vi "main.vi"() -> ()   [LabVIEW 2020]
uses:
  Typedef/QueueOperation.ctl
  Typedef/TimeCluster.ctl
  Strict Type Def/LowBean.ctl
  Strict Type Def/LowMilk.ctl
  Strict Type Def/Chamber.ctl
  Strict Type Def/Dispenser.ctl
  Strict Type Def/Low Water.ctl
  Strict Type Def/Purging.ctl
  Strict Type Def/Heating.ctl
  Strict Type Def/Grinding.ctl
  Strict Type Def/Brewing.ctl
  Strict Type Def/Dispensing.ctl
  Typedef/DataCluster.ctl
  <vilib>/Utility/config.llb/NI_LVConfig.lvlib
panel:
  out "error out":errorcluster
  in  "error in (no error)":errorcluster
  in  "Power":bool
  out "Total Cups":i32
  out "Elapsed Time":dbl
  out "Dispensing":T1
  out "Brewing":T2
  out "Grinding":T3
  out "Heating":T4
  out "Purging":T5
  out "Dispenser":T6 scale=0.0..60.0
  out "Chamber":T7 scale=0.0..60.0
  out "Low Milk":T8
  out "Low Bean":T9
  out "Low Water":T10
  out "Milk Level":i32(slide) min=0 max=100 scale=0.0..100.0
  out "Bean Level":i32(slide) min=0 max=100 scale=0.0..100.0
  out "Water Level":i32(slide) min=0 max=100 scale=0.0..100.0
  in  "Type":i32(knob) scale=0.0..2.0
  in  "Carafe":bool
  in  "Cup":bool
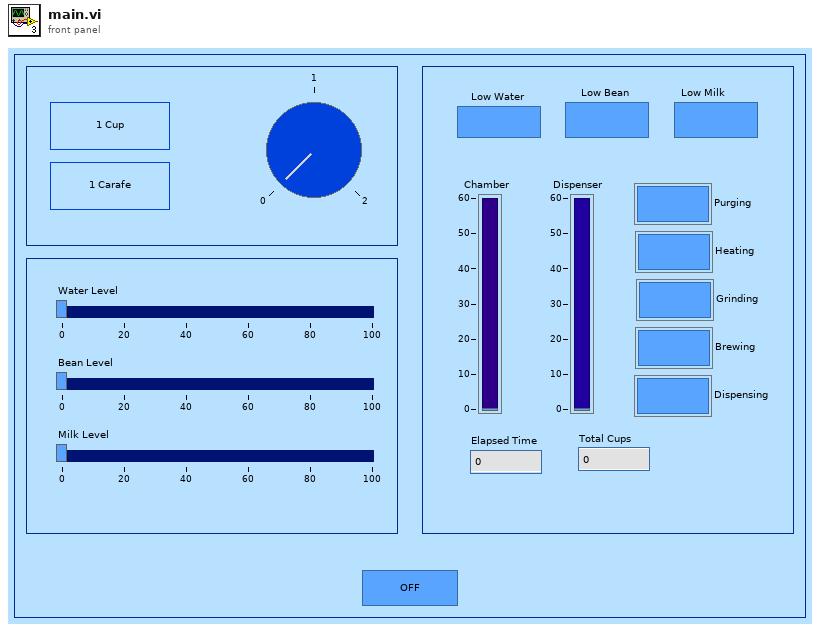
[diagram p1: front panel]
types:
  T1 = typedef "Dispensing.ctl" = bool
  T2 = typedef "Brewing.ctl" = bool
  T3 = typedef "Grinding.ctl" = bool
  T4 = typedef "Heating.ctl" = bool
  T5 = typedef "Purging.ctl" = bool
  T6 = typedef "Dispenser.ctl" = u8
  T7 = typedef "Chamber.ctl" = u8
  T8 = typedef "LowMilk.ctl" = bool
  T9 = typedef "LowBean.ctl" = bool
  T10 = typedef "Low Water.ctl" = bool
  T11 = typedef "DataCluster.ctl" = cluster{"Cup":bool, "Type":i32, "Carafe":bool, "Bean Level":i32, "Water Level":i32, "Milk Level":i32, "Low Bean":T9, "Low Milk":T8, "Chamber":T7, "Dispenser":T6, "Low Water":T10, "Elapsed Time":dbl, "Purging":T5, "Heating":T4, "Grinding":T3, "Brewing":T2, "Dispensing":T1, "Total Cups":i32, "Power":bool, "Timer":T12, "Path":path, "Shutdown":bool}
  T12 = typedef "TimeCluster.ctl" = cluster{"Relative time":dbl, "Initial Time":dbl, "Set Timer":i32, "Start/Stop":bool, "Pause/Resume":bool}
  T13 = typedef "QueueOperation.ctl" = enum16{"Create", "Enqueue", "Dequeue", "Flush", "Close"}
  T14 = enum8{"Enabled", "Disabled", "Disabled and Grayed Out"}
  T15 = typedef "NI_LVConfig.lvlib/Config Data RefNum.ctl" = refnum<k1>
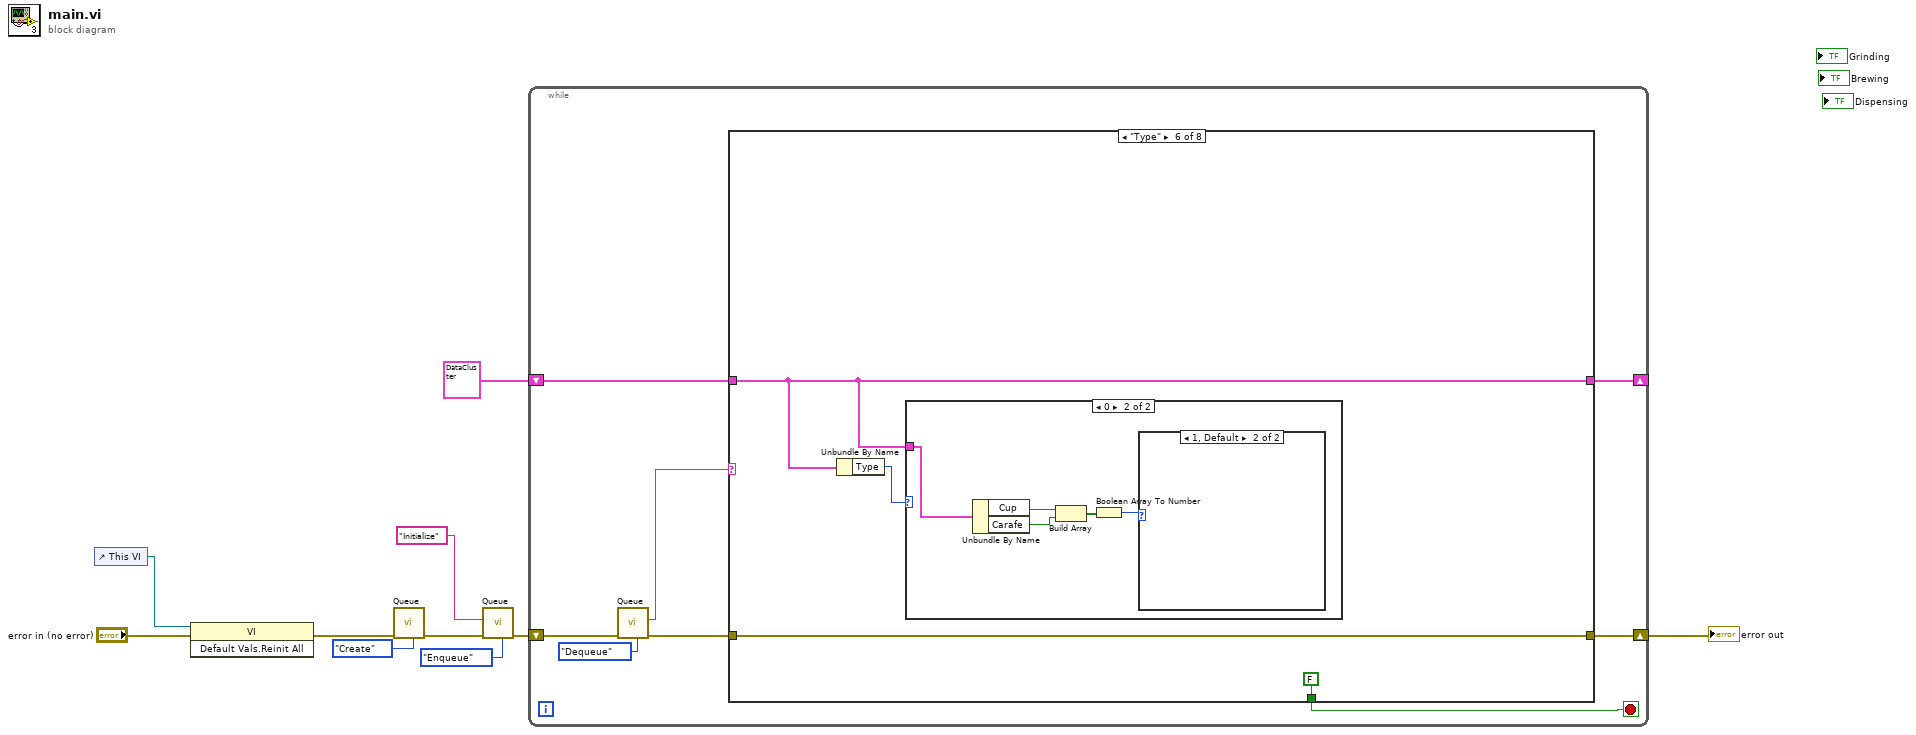
[diagram p0: block diagram]
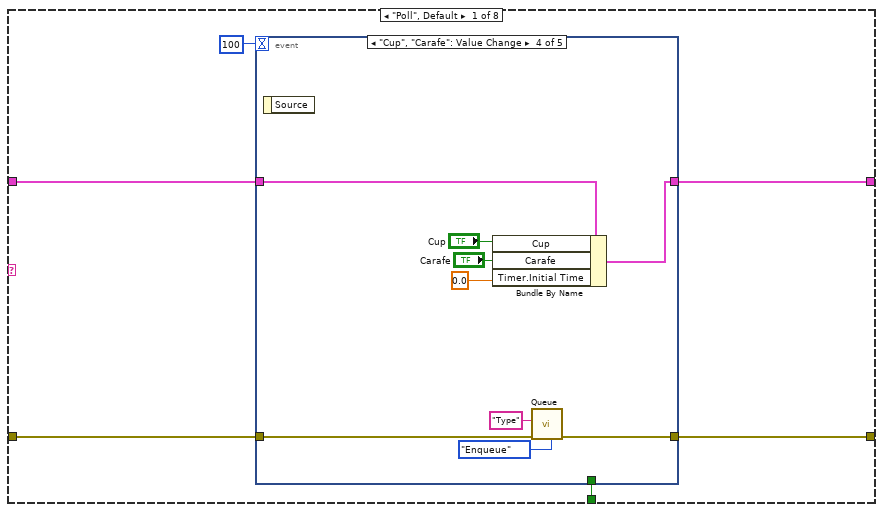
[diagram p2: hidden frame]
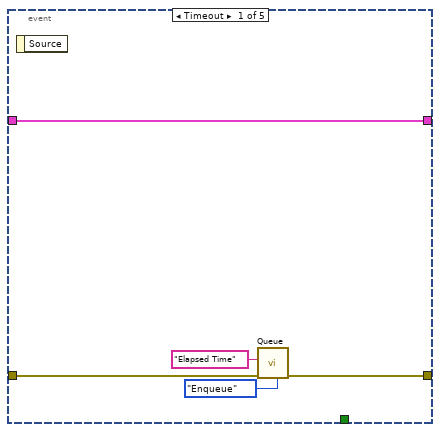
[diagram p3: hidden frame]
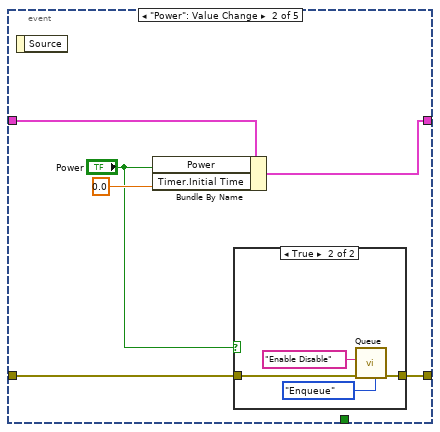
[diagram p4: hidden frame]
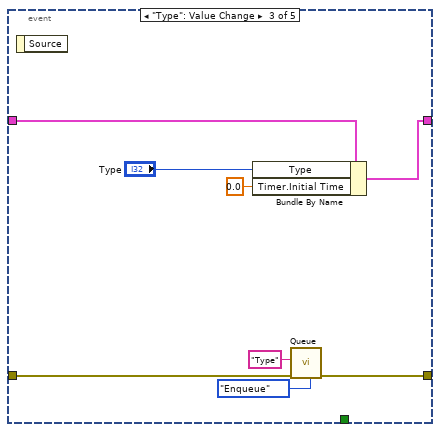
[diagram p6: hidden frame]
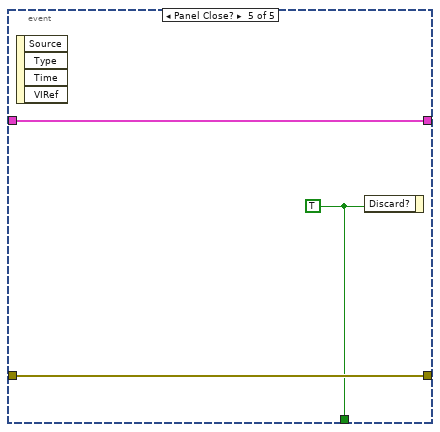
[diagram p7: hidden frame]
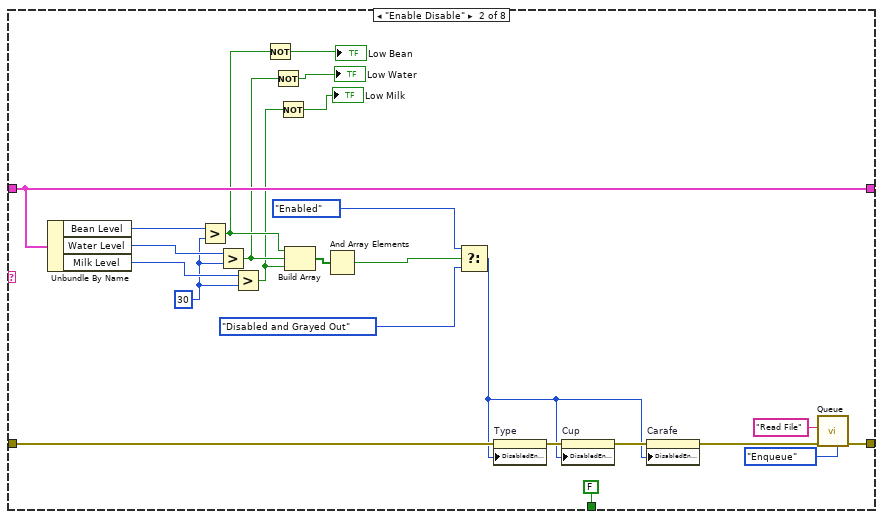
[diagram p8: hidden frame]
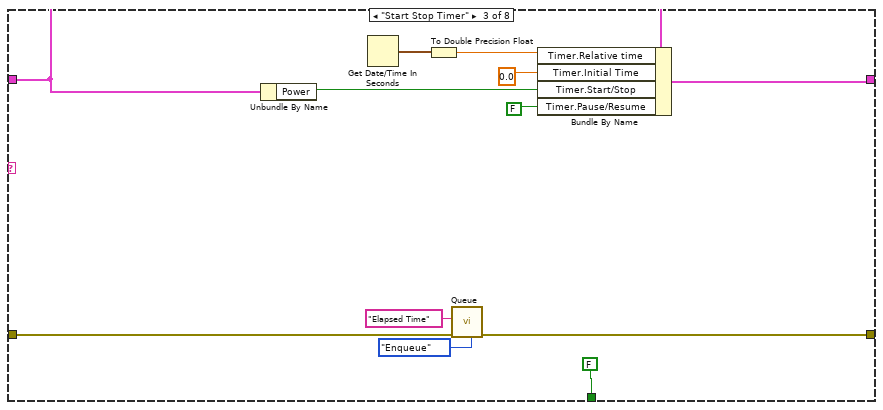
[diagram p9: hidden frame]
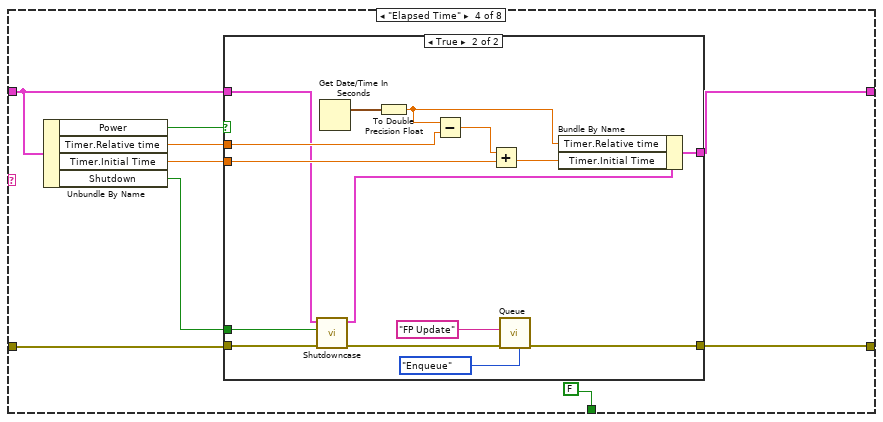
[diagram p10: hidden frame]
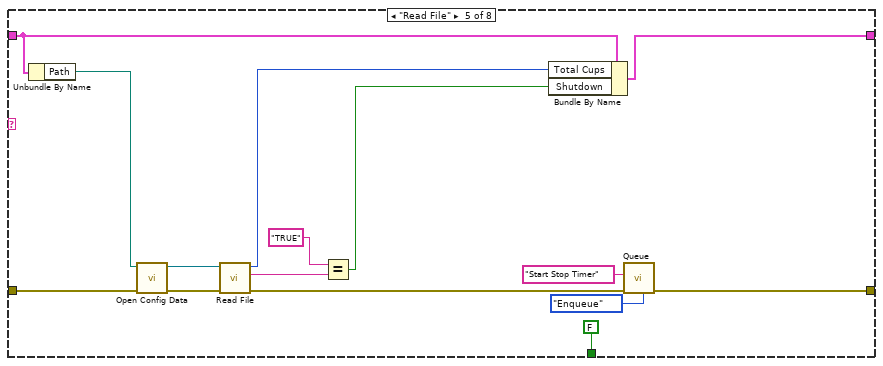
[diagram p12: hidden frame]
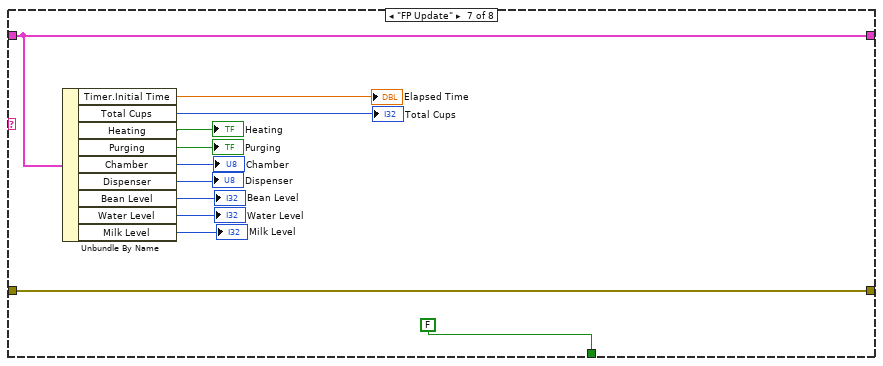
[diagram p15: hidden frame]
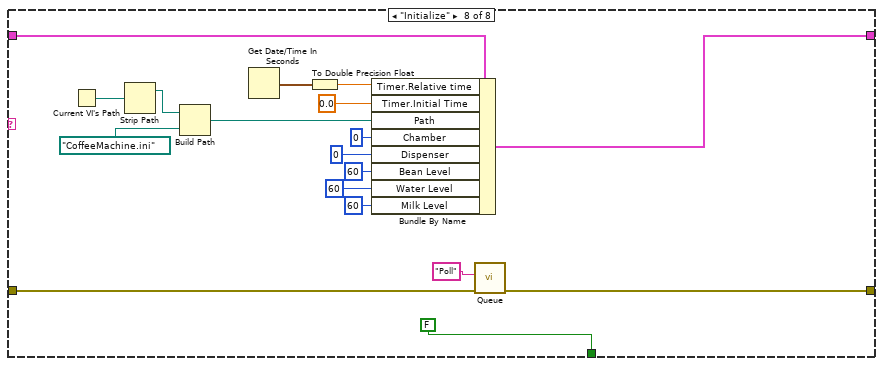
[diagram p16: hidden frame]
diagram:
  n1 = control-ref of="This VI"() -> (w8:refnum<vi>)
  n2 = invoke class="VI" method="Default Vals.Reinit All"(reference=w8, error in="error in (no error)") -> (error out=w7:errorcluster)  [unwired: 1 in, 2 out]
  n3 = call "Queue.vi"("Enum"=QueueOperation."Create", "error in (no error)"=w7) -> ("error out"=w5:errorcluster)  [unwired: 7 in, 2 out]
  n4 = call "Queue.vi"("Enum"=QueueOperation."Enqueue", "error in (no error)"=w5, "Enqueue Element"="Initialize") -> ("error out"=w4:errorcluster)  [unwired: 6 in, 2 out]
  n5 = while {
    shift-right: [w16] -> w9
    shift-left: w4 -> [w18]
    shift-right: [w13] -> _
    shift-left: T11 {"Cup"=FALSE, "Type"=0, "Carafe"=FALSE, "Bean Level"=0, "Water Level"=0, "Milk Level"=0, "Low Bean"=FALSE, "Low Milk"=FALSE, "Chamber"=1, "Dispenser"=1, "Low Water"=FALSE, "Elapsed Time"=0.0, "Purging"=FALSE, "Heating"=FALSE, "Grinding"=FALSE, "Brewing"=FALSE, "Dispensing"=FALSE, "Total Cups"=0, "Power"=FALSE, "Timer"={"Relative time"=0.0, "Initial Time"=0.0, "Set Timer"=0, "Start/Stop"=FALSE, "Pause/Resume"=FALSE}, "Path"=path "", "Shutdown"=FALSE} -> [w12]
    stop <- w11 stop-if-true
    n6 = call "Queue.vi"("Enum"=QueueOperation."Dequeue", "error in (no error)"=w18) -> ("error out"=w15:errorcluster, "Dequeued Element"=w14:string)  [unwired: 7 in, 1 out]
    n7 = case shown="\"Type\"" w14 {
      tunnel: [w24 w72 w87 w100 w125 w141 w158 w175] -> w16
      tunnel: w15 -> [w23 w84 w88 w99 w136 w141 w158 w176]
      tunnel: [w21 w82 w96 w101 w128 w138 w156 w171] -> w13
      tunnel: w12 -> [w20 w82 w90 w102 w129 w138 w156 w172]
      tunnel: [w19 FALSE FALSE FALSE FALSE FALSE FALSE FALSE] -> w11
      frame "Poll", Default {
        n8 = event shown="[3] \"Cup\", \"Carafe\": Value Change" {
          selector: _ -> [_ _ _ _ _]
          dyn-events: _ -> [_ _ _ _ _]
          timeout: 100 -> [_ _ _ _ _]
          tunnel: [w27 w32 w43 w52 w59] -> w24
          tunnel: w23 -> [w28 w33 w44 w53 w59]
          tunnel: [w29 w34 w47 w57 w60] -> w21
          tunnel: w20 -> [w29 w35 w48 w51 w60]
          tunnel: [_ _ _ _ w58] -> w19
          event Timeout {
            n9 = event-data() -> ()  [unwired: 1 in, 1 out]
            n10 = call "Queue.vi"("Enum"=QueueOperation."Enqueue", "error in (no error)"=w28, "Enqueue Element"="Elapsed Time") -> ("error out"=w27:errorcluster)  [unwired: 6 in, 2 out]
          }
          event "Power": Value Change {
            n11 = event-data() -> ()  [unwired: 1 in, 1 out]
            n12 = Bundle By Name(cluster=w35, "Power"="Power", "Timer.Initial Time"=0.0) -> (w34:T11)
            n13 = case shown="True" "Power" {
              tunnel: w33 -> [w36 w40]
              tunnel: [w36 w39] -> w32
              frame False {
              }
              frame True {
                n14 = call "Queue.vi"("Enum"=QueueOperation."Enqueue", "error in (no error)"=w40, "Enqueue Element"="Enable Disable") -> ("error out"=w39:errorcluster)  [unwired: 6 in, 2 out]
              }
            }
          }
          event "Type": Value Change {
            n15 = event-data() -> ()  [unwired: 1 in, 1 out]
            n16 = Bundle By Name(cluster=w48, "Type"="Type", "Timer.Initial Time"=0.0) -> (w47:T11)
            n17 = call "Queue.vi"("Enum"=QueueOperation."Enqueue", "error in (no error)"=w44, "Enqueue Element"="Type") -> ("error out"=w43:errorcluster)  [unwired: 6 in, 2 out]
          }
          event "Cup", "Carafe": Value Change {
            n18 = event-data() -> ()  [unwired: 1 in, 1 out]
            n19 = Bundle By Name(cluster=w51, "Cup"="Cup", "Carafe"="Carafe", "Timer.Initial Time"=0.0) -> (w57:T11)
            n20 = call "Queue.vi"("Enum"=QueueOperation."Enqueue", "error in (no error)"=w53, "Enqueue Element"="Type") -> ("error out"=w52:errorcluster)  [unwired: 6 in, 2 out]
          }
          event Panel Close? {
            w58 = TRUE
            n21 = event-data() -> ()  [unwired: 1 in, 4 out]
            n22 = event-data("Discard?"=w58) -> ()  [unwired: 1 in, 1 out]
          }
        }
      }
      frame "Enable Disable" {
        w78 = 30
        n23 = Unbundle By Name(w82) -> ("Bean Level"=w81:i32, "Water Level"=w80:i32, "Milk Level"=w79:i32)
        n24 = Greater?(x=w81, y=w78) -> (0:w65:bool)
        n25 = Greater?(x=w80, y=w78) -> (0:w63:bool)
        n26 = Greater?(x=w79, y=w78) -> (0:w61:bool)
        n27 = Not(x=w65) -> (.not. x?=→"Low Bean":bool)
        n28 = Not(x=w63) -> (.not. x?=→"Low Water":bool)
        n29 = Not(x=w61) -> (.not. x?=→"Low Milk":bool)
        n30 = Build Array(w65, w63, w61) -> (w77:bool[])
        n31 = And Array Elements(Boolean array=w77) -> (logical AND=w76:bool)
        n32 = Select(t=T14."Enabled" ("Disabled"), s=w76, f=T14."Disabled and Grayed Out" ("Disabled")) -> (s? t:f=w67:T14)
        n33 = property on="Type" class="Knob (strict)"(error in=w84, "DisabledEnum"=w67) -> (error out=w73:errorcluster)  [unwired: 1 in, 1 out]
        n34 = property on="Cup" class="Bool"(error in=w73, "DisabledEnum"=w67) -> (error out=w69:errorcluster)  [unwired: 1 in, 1 out]
        n35 = property on="Carafe" class="Bool"(error in=w69, "DisabledEnum"=w67) -> (error out=w68:errorcluster)  [unwired: 1 in, 1 out]
        n36 = call "Queue.vi"("Enum"=QueueOperation."Enqueue", "error in (no error)"=w68, "Enqueue Element"="Read File") -> ("error out"=w72:errorcluster)  [unwired: 6 in, 2 out]
      }
      frame "Start Stop Timer" {
        n37 = Unbundle By Name(w90) -> ("Power"=w89:bool)
        n38 = Get Date/Time In Seconds() -> (seconds since 1Jan1904=w95:timestamp)
        n39 = To Double Precision Float(number=w95) -> (double precision float=w94:dbl)
        n40 = call "Queue.vi"("Enum"=QueueOperation."Enqueue", "error in (no error)"=w88, "Enqueue Element"="Elapsed Time") -> ("error out"=w87:errorcluster)  [unwired: 6 in, 2 out]
        n41 = Bundle By Name(cluster=w90, "Timer.Relative time"=w94, "Timer.Initial Time"=0.0, "Timer.Start/Stop"=w89, "Timer.Pause/Resume"=FALSE) -> (w96:T11)
      }
      frame "Elapsed Time" {
        n42 = Unbundle By Name(w102) -> ("Power"=w98:bool, "Timer.Relative time"=w104:dbl, "Timer.Initial Time"=w103:dbl, "Shutdown"=w97:bool)
        n43 = case shown="True" w98 {
          tunnel: w104 -> [_ w122]
          tunnel: w103 -> [_ w121]
          tunnel: w102 -> [w107 w109]
          tunnel: [w107 w120] -> w101
          tunnel: [w106 w119] -> w100
          tunnel: w99 -> [w106 w116]
          tunnel: w97 -> [_ w110]
          frame False {
          }
          frame True {
            n44 = call "Shutdowncase.vi"("error in (no error)"=w116, "Boolean"=w110, "Data Cluster"=w109) -> ("error out"=w115:errorcluster, "output cluster"=w108:T11)  [unwired: 7 in]
            n45 = Get Date/Time In Seconds() -> (seconds since 1Jan1904=w114:timestamp)
            n46 = To Double Precision Float(number=w114) -> (double precision float=w112:dbl)
            n47 = Subtract(x=w112, y=w122) -> (x-y=w113:dbl)
            n48 = Add(x=w113, y=w121) -> (x+y=w111:dbl)
            n49 = call "Queue.vi"("Enum"=QueueOperation."Enqueue", "error in (no error)"=w115, "Enqueue Element"="FP Update") -> ("error out"=w119:errorcluster)  [unwired: 6 in, 2 out]
            n50 = Bundle By Name(cluster=w108, "Timer.Relative time"=w112, "Timer.Initial Time"=w111) -> (w120:T11)
          }
        }
      }
      frame "Read File" {
        n51 = Unbundle By Name(w129) -> ("Path"=w135:path)
        n52 = call <vilib>:"Open Config Data.vi"("error in (no error)"=w136, "configuration file path"=w135) -> ("error out"=w134:errorcluster, "refnum"=w133:T15)  [unwired: 7 in, 1 out]
        n53 = call "Read File.vi"("error in (no error)"=w134, "Refnum in"=w133) -> ("error out"=w126:errorcluster, "value"=w132:string, "value 2"=w130:i32)  [unwired: 7 in]
        n54 = Equal?(x="TRUE", y=w132) -> (x = y?=w127:bool)
        n55 = Bundle By Name(cluster=w129, "Total Cups"=w130, "Shutdown"=w127) -> (w128:T11)
        n56 = call "Queue.vi"("Enum"=QueueOperation."Enqueue", "error in (no error)"=w126, "Enqueue Element"="Start Stop Timer") -> ("error out"=w125:errorcluster)  [unwired: 6 in, 2 out]
      }
      frame "Type" {
        n57 = Unbundle By Name(w138) -> ("Type"=w139:i32)
        n58 = case shown="0" w139 {
          tunnel: w138 -> [_ w146]
          frame 0, Default {
          }
          frame 0 {
            n59 = Unbundle By Name(w146) -> ("Cup"=w145:bool, "Carafe"=w144:bool)
            n60 = Build Array(w145, w144) -> (w143:bool[])
            n61 = Boolean Array To Number(Boolean array=w143) -> (number=w142:u32)
            n62 = case shown="1, Default" w142 {
              frame 0 {
              }
              frame 1, Default {
              }
            }
          }
        }
      }
      frame "FP Update" {
        n63 = Unbundle By Name(w156) -> ("Timer.Initial Time"=→"Elapsed Time":dbl, "Total Cups"=→"Total Cups":i32, "Heating"=→"Heating":T4, "Purging"=→"Purging":T5, "Chamber"=→"Chamber":T7, "Dispenser"=→"Dispenser":T6, "Bean Level"=→"Bean Level":i32, "Water Level"=→"Water Level":i32, "Milk Level"=→"Milk Level":i32)
      }
      frame "Initialize" {
        n64 = Current VI's Path() -> (path=w167:path)
        n65 = Strip Path(path=w167) -> (stripped path=w166:path)  [unwired: 1 out]
        n66 = Build Path(base path=w166, name or relative path=path "CoffeeMachine.ini") -> (appended path=w164:path)
        n67 = Get Date/Time In Seconds() -> (seconds since 1Jan1904=w170:timestamp)
        n68 = To Double Precision Float(number=w170) -> (double precision float=w169:dbl)
        n69 = Bundle By Name(cluster=w172, "Timer.Relative time"=w169, "Timer.Initial Time"=0.0, "Path"=w164, "Chamber"=T7 0, "Dispenser"=T6 0, "Bean Level"=60, "Water Level"=60, "Milk Level"=60) -> (w171:T11)
        n70 = call "Queue.vi"("error in (no error)"=w176, "Enqueue Element"="Poll") -> ("error out"=w175:errorcluster)  [unwired: 7 in, 2 out]
      }
    }
  }
  "error out" <- w9
